vi "Generate Waveform.vi"(8 "error in (no error)":errorcluster, 11 "Waveform in":refnum<class "Advanced Waveform.lvclass">) -> (0 "error out":errorcluster, 3 "Waveform out":refnum<class "Advanced Waveform.lvclass">)   [LabVIEW 2011, in "Advanced Waveform.lvclass"]
uses:
  Advanced Waveform.lvclass
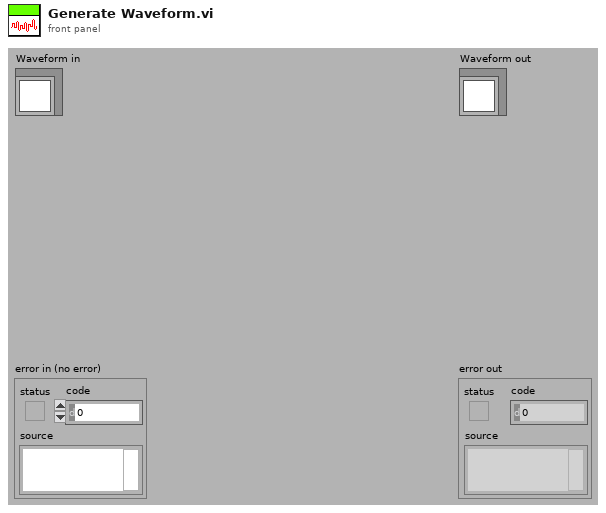
[diagram p1: front panel]
types:
  T1 = typedef "Waveform Type.ctl" = enum16{"Sine", "Square", "Triangle"}
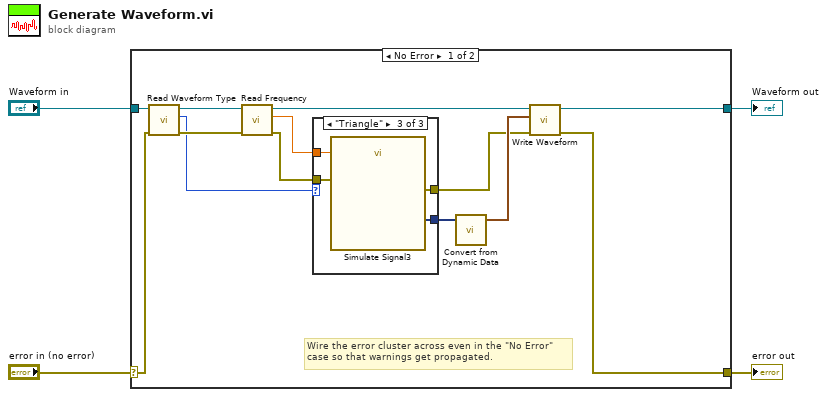
[diagram p0: block diagram]
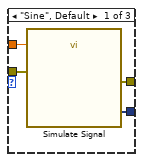
[diagram p2: hidden frame]
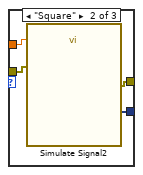
[diagram p3: hidden frame]
diagram:
  n1 = case shown="No Error" "error in (no error)" {
    selector: "error in (no error)" -> [w6 w31]
    tunnel: [w10 w31] -> w3
    tunnel: [w11 w30] -> w1
    tunnel: "Waveform in" -> [w9 w30]
    frame No Error {
      # "Wire the error cluster across even in the \"No Error\"\ncase so that warnings get propagated."
      n2 = call-dynamic "Read Waveform Type.vi"("error in (no error)"=w6, "Advanced Waveform in"=w9) -> ("error out"=w7:errorcluster, "Waveform Type"=w5:T1, "Advanced Waveform out"=w8:refnum<class "Advanced Waveform.lvclass">)  [unwired: 7 in]
      n3 = call-dynamic "Read Frequency.vi"("error in (no error)"=w7, "Waveform in"=w8) -> ("error out"=w15:errorcluster, "Frequency"=w17:dbl, "Waveform out"=w14:refnum<class "Advanced Waveform.lvclass">)  [unwired: 7 in]
      n4 = case shown="\"Triangle\"" w5 {
        tunnel: w17 -> [w21 w25 w29]
        tunnel: [w20 w24 w28] -> w16
        tunnel: w15 -> [w19 w23 w27]
        tunnel: [w18 w22 w26] -> w12
        frame "Sine", Default {
          n5 = call "Simulate Signal"("Frequency"=w21, "error in (no error)"=w19) -> ("Sine"=w20:dynamicdata, "error out"=w18:errorcluster)  [unwired: 12 in]
        }
        frame "Square" {
          n6 = call "Simulate Signal2"("Frequency"=w25, "error in (no error)"=w23) -> ("Square"=w24:dynamicdata, "error out"=w22:errorcluster)  [unwired: 12 in]
        }
        frame "Triangle" {
          n7 = call "Simulate Signal3"("Frequency"=w29, "error in (no error)"=w27) -> ("Triangle"=w28:dynamicdata, "error out"=w26:errorcluster)  [unwired: 12 in]
        }
      }
      n8 = call "Convert from Dynamic Data"("Dynamic Data Type"=w16) -> ("Waveform"=w13:waveform(dbl))  [unwired: 3 in]
      n9 = call-dynamic "Write Waveform.vi"("error in (no error)"=w12, "Waveform"=w13, "Waveform in"=w14) -> ("error out"=w10:errorcluster, "Waveform out"=w11:refnum<class "Advanced Waveform.lvclass">)  [unwired: 7 in]
    }
    frame Error {
    }
  }
  "error out" <- w3
  "Waveform out" <- w1
